vi "test - Complex.vi"(8 "error in (no error)":errorcluster, 11 "TestCase in":refnum<class "testcase-Supported-Datatype.lvclass">) -> (0 "error out":errorcluster, 3 "TestCase out":refnum<class "testcase-Supported-Datatype.lvclass">)   [LabVIEW 2017, in "testcase-Supported-Datatype.lvclass"]
uses:
  testcase-Supported-Datatype.lvclass
  b68c48f3-9af3-4157-b5ae-59a6d9f15f68.vi
  e37f20e3-ff9d-4038-9bc4-cee086f65af6.vi
  addons/API-String-Arugments-Support/_Support/Data To API String Arguments.vi
  addons/API-String-Arugments-Support/_Support/Convert API String Arguments to Data(variant).vi
  <vilib>/addons/_JKI Toolkits/VI Tester/TestCase.llb/TestCase.lvclass
  C:/Program Files (x86)/National Instruments/LabVIEW 2017/vi.lib/addons/_JKI Toolkits/VI Tester/TestCase.llb/TestCase.lvclass
panel:
  out "resulting string":string
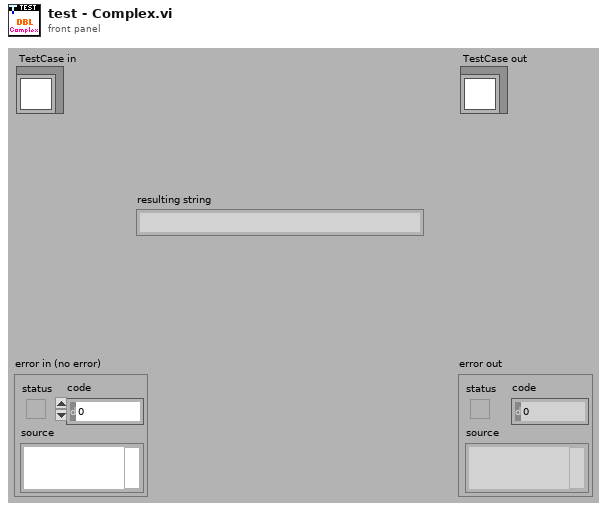
[diagram p1: front panel]
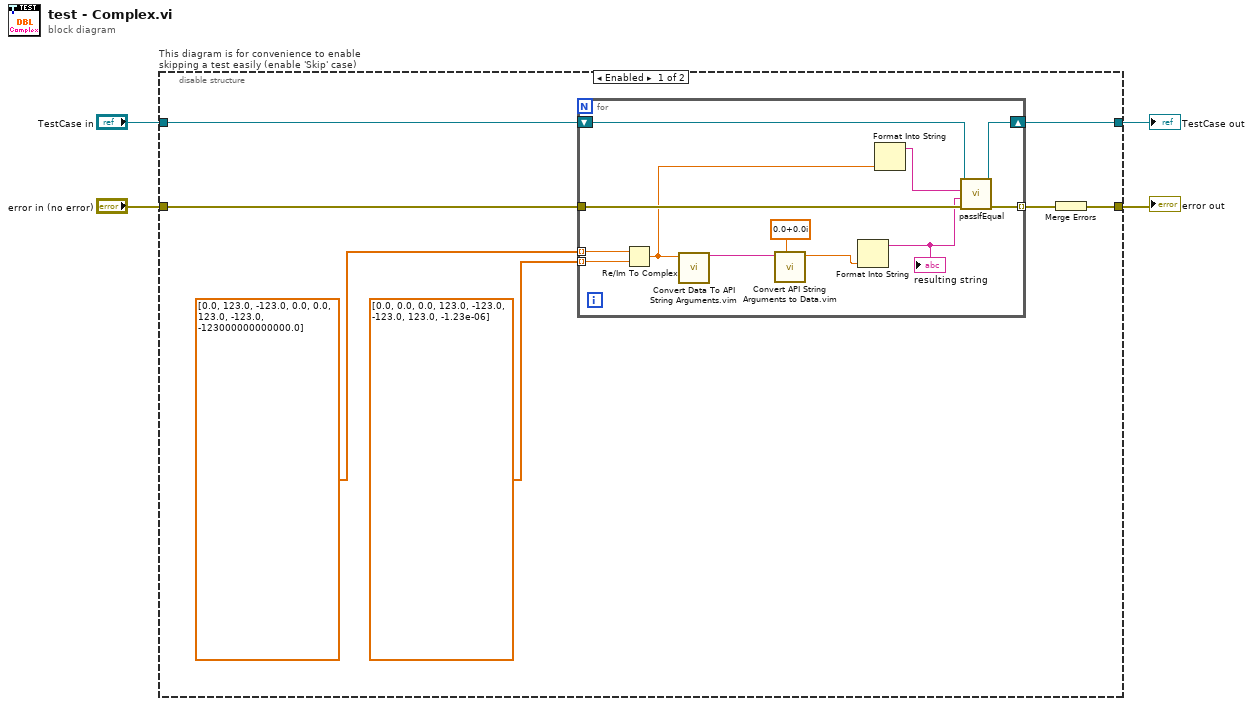
[diagram p0: block diagram]
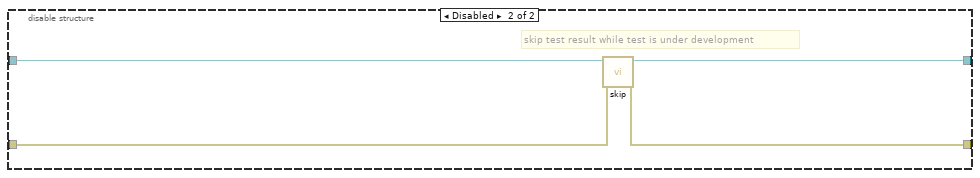
[diagram p2: hidden frame]
diagram:
  n1 = disable-structure "This diagram is for convenience to enable skipping a test easily (enable 'Skip' case)" shown="Enabled" {
    disable-tunnel: "TestCase in" -> [w11 w27]
    disable-tunnel: [w6 w25] -> w1
    disable-tunnel: [w5 w26] -> w3
    disable-tunnel: "error in (no error)" -> [w10 w24]
    frame Enabled {
      n2 = for {
        tunnel: w10 -> [w22]
        tunnel: dbl[] [0.0, 123.0, -123.0, 0.0, 0.0, 123.0, -123.0, -123000000000000.0] ("x") -> [w20] mode=indexing
        tunnel: dbl[] [0.0, 0.0, 0.0, 123.0, -123.0, -123.0, 123.0, -1.23e-06] ("x") -> [w18] mode=indexing
        shift-right: [w17] -> w6
        shift-left: w11 -> [w23]
        tunnel: [w16] -> w7 mode=indexing
        n3 = Re/Im To Complex(1:w18, 2:w20) -> (0:w15:cdb)
        n4 = call "Convert Data To API String Arguments.vim"("Data"=w15) -> ("API String"=w21:string)  [unwired: 7 in, 1 out]
        n5 = call "Convert API String Arguments to Data.vim"("Reference Type"=cdb 0.0+0.0i ("x + iy"), "API String"=w21) -> ("Data"=w13:cdb)  [unwired: 6 in, 1 out]
        n6 = Format Into String(w13) -> (resulting string=w12:string)  [unwired: 3 in, 1 out]
        "resulting string" <- w12
        n7 = Format Into String(w15) -> (resulting string=w14:string)  [unwired: 3 in, 1 out]
        n8 = call-dynamic "passIfEqual.vi"("error in (no error)"=w22, "y"=w12, "x"=w14, "TestCase in"=w23) -> ("error out"=w16:errorcluster, "TestCase out"=w17:refnum<class "testcase-Supported-Datatype.lvclass">)  [unwired: 6 in]
      }
      n9 = Merge Errors(w7) -> (w5:errorcluster)
    }
    frame Disabled {
      # "skip test result while test is under development"
      n10 = call <vilib>:"skip.vi"("error in (no error)"=w24, "TestCase in"=w27) -> ("error out"=w26:errorcluster, "TestCase out"=w25:refnum<class "testcase-Supported-Datatype.lvclass">)  [unwired: 8 in]
    }
  }
  "error out" <- w3
  "TestCase out" <- w1
